vi "Polling Core.vi"(8 "Error In":errorcluster, 11 "CS++TestMotor in":refnum<class "CS++TestMotor.lvclass">) -> (0 "Error Out":errorcluster, 3 "CS++TestMotor out":refnum<class "CS++TestMotor.lvclass">)   [LabVIEW 2015, in "CS++TestMotor.lvlib" / "CS++TestMotor.lvclass"]
doc: "Implement the pseudo-periodic action in your override.vi."
uses:
  CS++TestMotor.lvclass
  CS++TestMotor.lvclass/CS++TestMotor.ctl
  CSPP_DeviceBase/CS++Motor Messages/Move Msg/Move Msg.lvclass/Move Msg.ctl
  <vilib>/ActorFramework/Message Enqueuer/Message Enqueuer.lvclass/Message Enqueuer.ctl
  CSPP_DeviceBase/CS++Motor Messages/ReferenceMove Msg/ReferenceMove Msg.lvclass/ReferenceMove Msg.ctl
  <vilib>/ActorFramework/Message Enqueuer/Enqueue.vi
  <vilib>/ActorFramework/Message Priority Queue/Priority Enqueue.vi
  CSPP_DeviceBase/CS++Motor Messages/Move Msg/Move Msg.lvclass
  CSPP_DeviceBase/CS++Motor Messages/ReferenceMove Msg/ReferenceMove Msg.lvclass
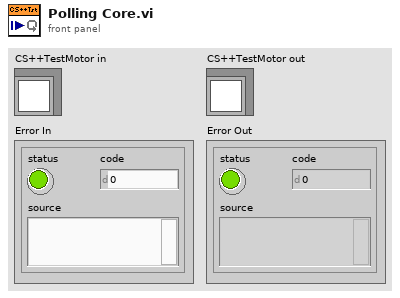
[diagram p1: front panel]
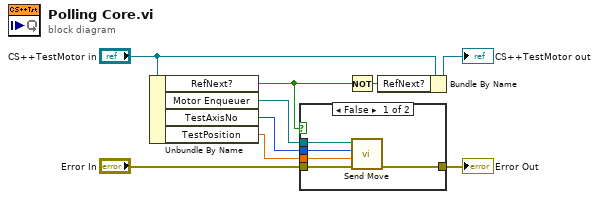
[diagram p0: block diagram]
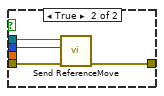
[diagram p2: hidden frame]
diagram:
  n1 = Unbundle By Name("CS++TestMotor in") -> ("RefNext?"=w6:bool, "Motor Enqueuer"=w5:refnum<class "Message Enqueuer.lvclass">, "TestAxisNo"=w1:u8, "TestPosition"=w2:dbl)
  n2 = case shown="False" w6 {
    tunnel: w5 -> [w12 w18]
    tunnel: "Error In" -> [w14 w17]
    tunnel: [w13 w16] -> w3
    tunnel: w2 -> [w11 _]
    tunnel: w1 -> [w10 w15]
    frame False {
      n3 = call "Send Move.vi"("error in (no error)"=w14, "Position"=w11, "AxisNumber"=w10, "Message Enqueuer"=w12) -> ("error out"=w13:errorcluster)  [unwired: 6 in, 1 out]
    }
    frame True {
      n4 = call "Send ReferenceMove.vi"("error in (no error)"=w17, "AxisNumber"=w15, "Message Enqueuer"=w18) -> ("error out"=w16:errorcluster)  [unwired: 7 in, 1 out]
    }
  }
  "Error Out" <- w3
  n5 = Not(x=w6) -> (.not. x?=w7:bool)
  n6 = Bundle By Name(cluster="CS++TestMotor in", "RefNext?"=w7) -> (→"CS++TestMotor out":refnum<class "CS++TestMotor.lvclass">)
